vi "Result Helper.vi"(9 "State":T1, 11 "Value In":refnum<class>) -> (0 "Error":errorcluster, 3 "Value":refnum<class>)   [LabVIEW 2020, in "Promises.lvlib" / "Future.lvclass"]
uses:
  Future.lvclass
  Result State.ctl
  Error Result/Error Result.lvclass
  Error Result/Error Result.lvclass/Error Result.ctl
  Future.lvclass/Future.ctl
  Promises.lvlib
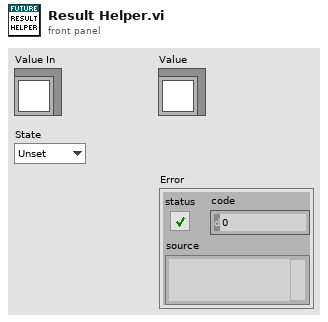
[diagram p1: front panel]
types:
  T1 = typedef "Promises.lvlib/Result State.ctl" = enum16{"Unset", "Error", "Success"}
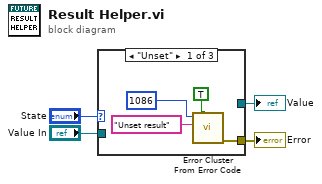
[diagram p0: block diagram]
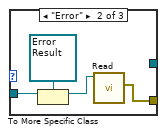
[diagram p2: hidden frame]
diagram:
  n1 = case shown="\"Unset\"" "State" {
    tunnel: "Value In" -> [_ w12 w13]
    tunnel: [w8 w9 _] -> w1
    tunnel: [_ _ w13] -> w2
    frame "Unset" {
      n2 = call <vilib>:"Error Cluster From Error Code.vi"("show call chain? (False)"=TRUE, "error message (\"\")"="Unset result" ("error message (\"\")"), "error code (0)"=1086) -> ("error out"=w8:errorcluster)  [unwired: 6 in]
    }
    frame "Error" {
      n3 = To More Specific Class(target class=refnum<class "Error Result.lvclass"> refnum ("Futures:Error Result.lvclass"), reference=w12) -> (specific class reference=w10:refnum<class "Error Result.lvclass">)  [unwired: 1 in, 1 out]
      n4 = call "Read.vi"("Error Result in"=w10) -> ("Error"=w9:errorcluster)  [unwired: 10 in]
    }
    frame "Success" {
    }
  }
  "Value" <- w2
  "Error" <- w1
